vi "Prepend Size.vi"(1 "data":string) -> (0 "data with size":string)   [LabVIEW 2015]
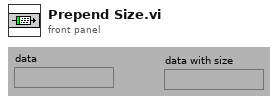
[diagram p1: front panel]
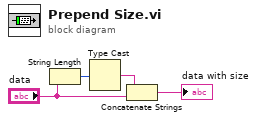
[diagram p0: block diagram]
diagram:
  n1 = String Length(string="data") -> (length=w1:i32)
  n2 = Type Cast(x=w1) -> (*(type *) &x=w3:string)  [unwired: 1 in]
  n3 = Concatenate Strings(w3, "data") -> (→"data with size":string)
